vi "DDS9954 Calibrate Microwave Power to Level Setting.vi"(4 "Desired Microwave Power [dBm]":dbl) -> (1 "Corresponding DDS Amplitude Fraction (0-1)":dbl)   [LabVIEW 2016]
uses:
  <vilib>/gmath/NI_Gmath.lvlib
panel:
  out "yi":dbl[](array[numeric]) format="%_6g"
  out "x*y":dbl
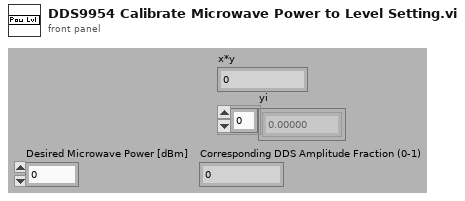
[diagram p1: front panel]
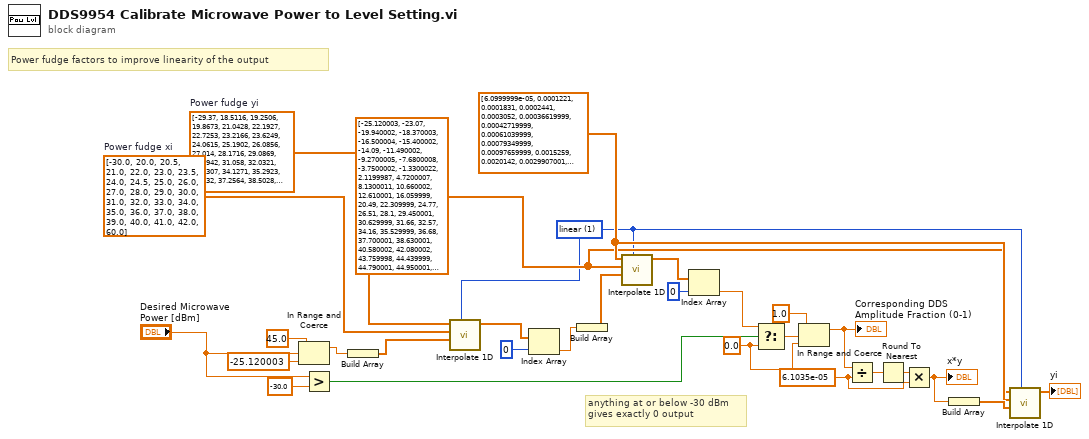
[diagram p0: block diagram]
diagram:
  w2 = dbl[] [-29.37, 18.5116, 19.2506, 19.8673, 21.0428, 22.1927, 22.7253, 23.2166, 23.6249, 24.0615, 25.1902, 26.0856, 27.014, 28.1716, 29.0869, 30.0942, 31.058, 32.0321, 33.0307, 34.1271, 35.2923, 36.132, 37.2564, 38.5028, 39.5528, 40.5755, 42.0, 60.0]  # Power fudge yi
  w1 = dbl[] [-30.0, 20.0, 20.5, 21.0, 22.0, 23.0, 23.5, 24.0, 24.5, 25.0, 26.0, 27.0, 28.0, 29.0, 30.0, 31.0, 32.0, 33.0, 34.0, 35.0, 36.0, 37.0, 38.0, 39.0, 40.0, 41.0, 42.0, 60.0]  # Power fudge xi
  w14 = 6.1035e-05 ("y")
  w10 = dbl[] [-25.120003, -23.07, -19.940002, -18.370003, -16.500004, -15.400002, -14.09, -11.490002, -9.2700005, -7.6800008, -3.7500002, -1.3300022, 2.1199987, 4.7200007, 8.1300011, 10.660002, 12.610001, 16.059999, 20.49, 22.309999, 24.77, 26.51, 28.1, 29.450001, 30.629999, 31.66, 32.57, 34.16, 35.529999, 36.68, 37.700001, 38.630001, 40.580002, 42.080002, 43.759998, 44.439999, 44.790001, 44.950001, 45.029999] ("subarray 2")
  w11 = dbl[] [6.0999999e-05, 0.0001221, 0.0001831, 0.0002441, 0.0003052, 0.00036619999, 0.00042719999, 0.00061039999, 0.00079349999, 0.00097659999, 0.0015259, 0.0020142, 0.0029907001, 0.0040282998, 0.0059814001, 0.0079955999, 0.0100098, 0.0150146, 0.025024399, 0.030029301, 0.039978001, 0.0499878, 0.059999999, 0.070006996, 0.080017, 0.090026997, 0.1, 0.12, 0.14, 0.16, 0.18000001, 0.2, 0.25, 0.30000001, 0.40000001, 0.5, 0.60000002, 0.69999999, 0.80000001] ("subarray")
  w23 = 0.0 ("f")
  w3 = 1 items=["nearest", "linear", "spline", "cubic Hermite", "Lagrange"] ("method")
  # "Power fudge factors to improve linearity of the output"
  # "anything at or below -30 dBm\ngives exactly 0 output"
  n1 = In Range and Coerce(upper limit=45.0, x="Desired Microwave Power [dBm]", lower limit=-25.120003) -> (coerced(x)=w21:dbl)  [unwired: 1 out]
  n2 = Greater?(x="Desired Microwave Power [dBm]", y=-30.0) -> (0:w27:bool)
  n3 = Build Array(w21) -> (w8:dbl[])
  n4 = call <vilib>:"Interpolate 1D.vi"("method"=w3, "xi"=w8, "X"=w1, "Y"=w2) -> ("yi"=w6:dbl[])  [unwired: 2 in, 5 out]
  n5 = Index Array(array=w6, index=0) -> (element=w5:dbl)
  n6 = Build Array(w5) -> (w4:dbl[])
  n7 = call <vilib>:"Interpolate 1D.vi"("method"=w3, "xi"=w4, "X"=w10, "Y"=w11) -> ("yi"=w29:dbl[])  [unwired: 2 in, 5 out]
  n8 = Index Array(array=w29, index=0) -> (element=w26:dbl)
  n9 = Select(t=w26, s=w27, f=w23) -> (s? t:f=w25:dbl)
  n10 = In Range and Coerce(upper limit=1.0, x=w25, lower limit=w23) -> (coerced(x)=w17:dbl)  [unwired: 1 out]
  "Corresponding DDS Amplitude Fraction (0-1)" <- w17
  n11 = Divide(x=w17, y=w14) -> (x/y=w16:dbl)
  n12 = Round To Nearest(number=w16) -> (nearest integer value=w15:dbl)
  n13 = Multiply(x=w15, y=w14) -> (x*y=w13:dbl)
  "x*y" <- w13
  n14 = Build Array(w13) -> (w12:dbl[])
  n15 = call <vilib>:"Interpolate 1D.vi"("method"=w3, "xi"=w12, "X"=w11, "Y"=w10) -> ("yi"=→"yi":dbl[])  [unwired: 2 in, 5 out]
